vi "Crop3DStack.vi"(10 "Crop Pixels":u16=30, 11 "3D Data":dbl[][][](array[numeric])) -> (3 "Cropped 3D Data":dbl[][][](array[numeric]))   [LabVIEW 2015]
panel:
  out "size(s) 2":i32[](array[numeric])
  out "size(s)":i32[](array[numeric])
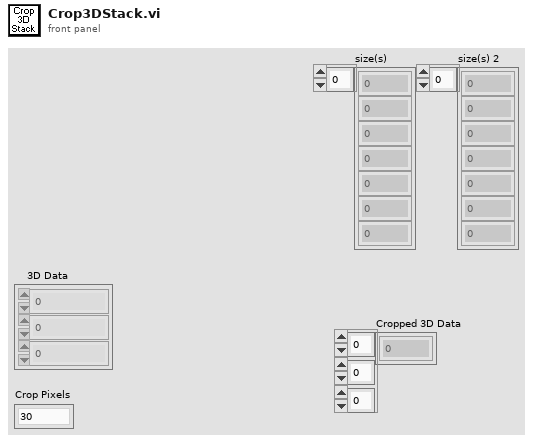
[diagram p1: front panel]
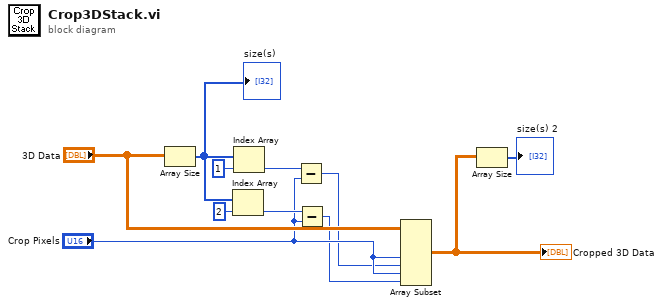
[diagram p0: block diagram]
diagram:
  n1 = Array Size(array="3D Data") -> (size(s)=w11:i32[])
  "size(s)" <- w11
  n2 = Index Array(array=w11, index=2) -> (element=w7:i32)
  n3 = Index Array(array=w11, index=1) -> (element=w8:i32)
  n4 = Subtract(x=w8, y="Crop Pixels") -> (x-y=w2:i32)
  n5 = Subtract(x=w7, y="Crop Pixels") -> (x-y=w1:i32)
  n6 = Array Subset(array="3D Data", index (dim 1)="Crop Pixels", length (dim 1)=w2, index (dim 2)="Crop Pixels", length (dim 2)=w1) -> (w5:dbl[][][])  [unwired: 2 in]
  "Cropped 3D Data" <- w5
  n7 = Array Size(array=w5) -> (size(s)=→"size(s) 2":i32[])
